vi "network2.vi"() -> ()   [LabVIEW 2009]
uses:
  <vilib>/vision/NI_Vision_Development_Module.lvlib
panel:
  out "Cluster":T1
  out "Filtered Image":T2(plugin-control)
  in  "res/2":i32
  in  "Sample Rate":i32=3
  out "Input Image":T2(plugin-control)
  in  "Input File Path":path
  in  "Stop Checking":bool
  out "Size of Inputs":i32
  in  "Num Iters":i32=2000
  out "Final Error":dbl(graph)
  in  "Stop Training":bool
  out "New Hidden Weights":dbl[][](array[numeric])
  out "Hidden Error":dbl[](array[numeric])
  out "New Output Weights":dbl[](array[numeric])
  in  "Training Constant":dbl=1.0
  out "Final Error for Back Prop":dbl
  out "Target":dbl
  out "Output":dbl
  in  "Num Not":i32=5
  in  "Num Line":i32=5
  out "Inputs":dbl[](array[numeric])
  in  "Num Hidden Layer":i32=128
  in  "Num Inputs":i32=64
  in  "Function Hidden Layer":u16(ring) items=["Siqmoid", "Linear", "Sign"]
  in  "Function Final Layer":u16(ring) items=["Siqmoid", "Linear", "Sign"]
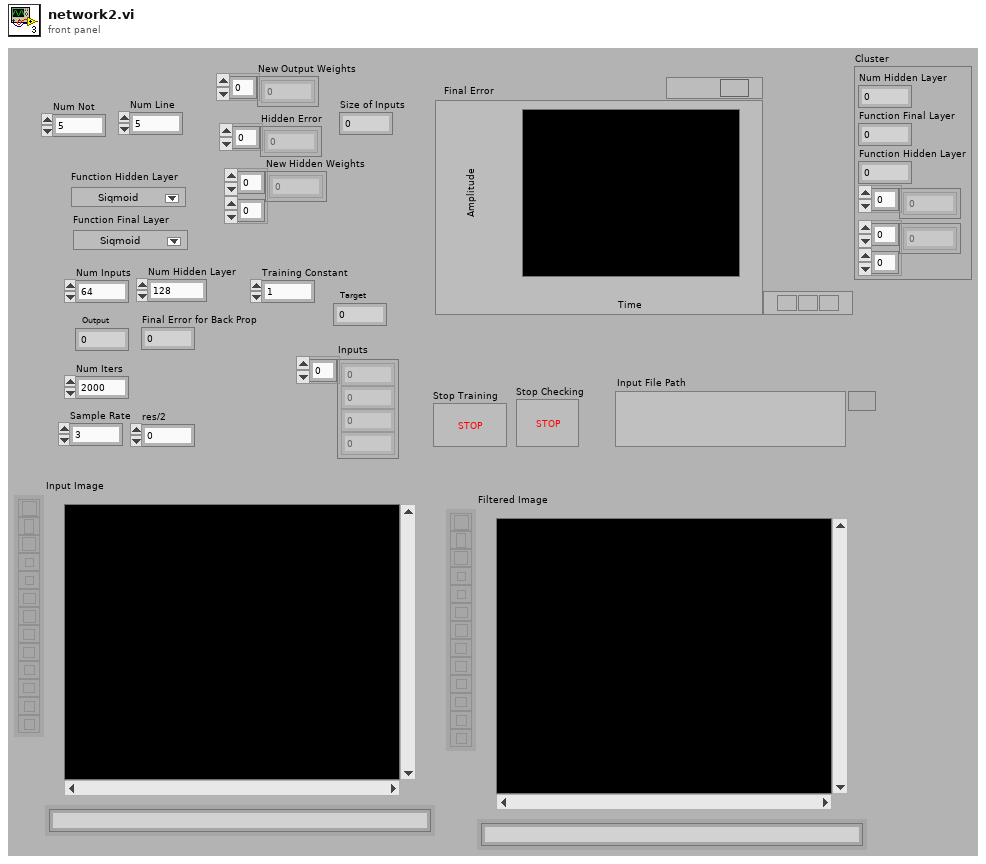
[diagram p1: front panel]
types:
  T1 = cluster{"Num Hidden Layer":i32, "Function Final Layer":u16, "Function Hidden Layer":u16, dbl[], dbl[][]}
  T2 = typedef "IMAQ Image.ctl" = refnum<image>
  T3 = typedef "Image Type" = u32
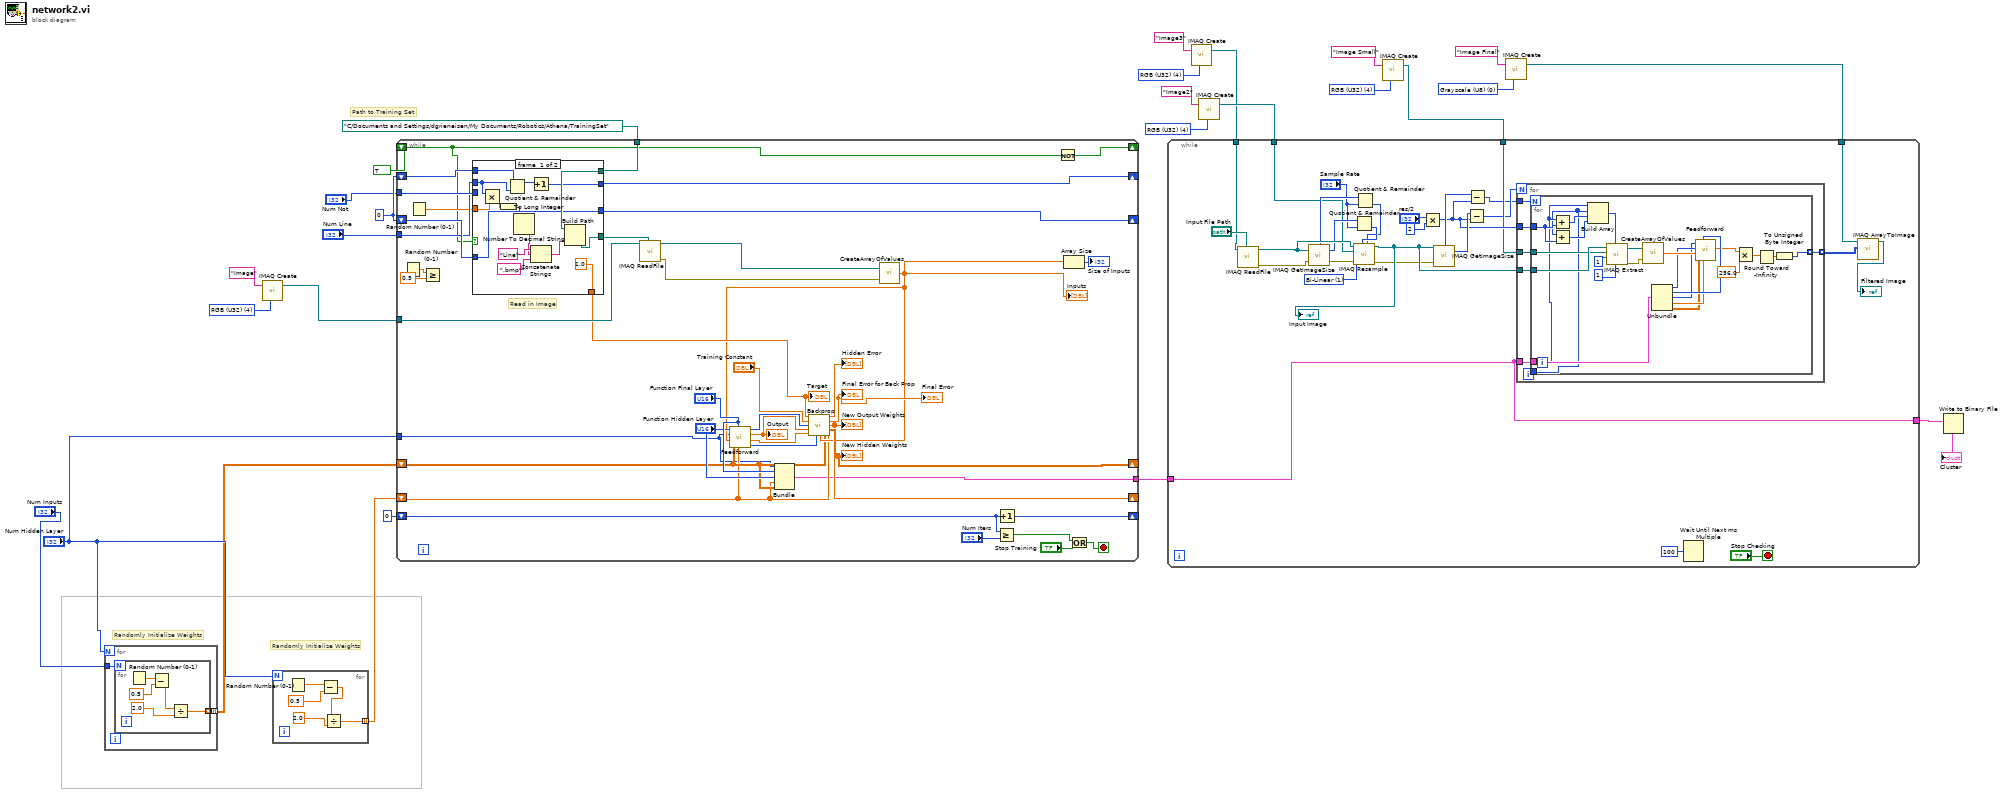
[diagram p0: block diagram]
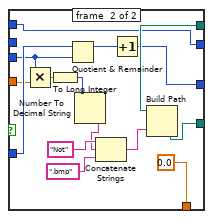
[diagram p2: hidden frame]
diagram:
  w4 = T3 4 items=["Grayscale (U8)", "Grayscale (I16)", "Grayscale (SGL)", "Complex (CSG)", "RGB (U32)", "HSL (U32)", "RGB (U64)", "Grayscale (U16)"] ("Image Type")
  w7 = T3 0 items=["Grayscale (U8)", "Grayscale (I16)", "Grayscale (SGL)", "Complex (CSG)", "RGB (U32)", "HSL (U32)", "RGB (U64)", "Grayscale (U16)"] ("Image Type")
  w11 = T3 4 items=["Grayscale (U8)", "Grayscale (I16)", "Grayscale (SGL)", "Complex (CSG)", "RGB (U32)", "HSL (U32)", "RGB (U64)", "Grayscale (U16)"] ("Image Type")
  w14 = T3 4 items=["Grayscale (U8)", "Grayscale (I16)", "Grayscale (SGL)", "Complex (CSG)", "RGB (U32)", "HSL (U32)", "RGB (U64)", "Grayscale (U16)"] ("Image Type")
  w21 = 0
  w25 = T3 4 items=["Grayscale (U8)", "Grayscale (I16)", "Grayscale (SGL)", "Complex (CSG)", "RGB (U32)", "HSL (U32)", "RGB (U64)", "Grayscale (U16)"] ("Image Type")
  # "Path to Training Set"
  # "Randomly Initialize Weights"
  # "Randomly Initialize Weights"
  n1 = for {
    N: "Num Hidden Layer" -> [_]
    tunnel: [w29] -> w22 mode=indexing
    tunnel: "Num Inputs" -> [w28]
    n2 = for {
      N: w28 -> [_]
      tunnel: [w30] -> w29 mode=indexing
      n3 = Random Number (0-1)() -> (number: 0 to 1=w31:dbl)
      n4 = Subtract(x=w31, y=0.5) -> (x-y=w33:dbl)
      n5 = Divide(x=w33, y=2.0) -> (x/y=w30:dbl)
    }
  }
  n6 = call "IMAQ Create"("Image Name"="Image", "Image Type"=w25) -> ("New Image"=w19:T2)  [unwired: 2 in, 2 out]
  n7 = for {
    N: "Num Hidden Layer" -> [_]
    tunnel: [w35] -> w23 mode=indexing
    n8 = Random Number (0-1)() -> (number: 0 to 1=w39:dbl)
    n9 = Subtract(x=w39, y=0.5) -> (x-y=w36:dbl)
    n10 = Divide(x=w36, y=2.0) -> (x/y=w35:dbl)
  }
  n11 = while {
    tunnel: "Num Hidden Layer" -> [w41]
    shift-right: [w73] -> _
    shift-left: w22 -> [w44]
    shift-right: [w72] -> _
    shift-left: w23 -> [w43]
    shift-right: [w52] -> _
    shift-left: w21 -> [w53]
    shift-right: [w55] -> _
    shift-left: w21 -> [w56]
    shift-right: [w71] -> _
    shift-left: TRUE -> [w40]
    tunnel: w19 -> [w70]
    tunnel: path "C:/Documents and Settings/dgrieneisen/My Documents/Robotics/Athena/TrainingSet" -> [w69]
    shift-right: [w60] -> _
    shift-left: 0 -> [w59]
    tunnel: "Num Not" -> [w57]
    tunnel: "Num Line" -> [w54]
    tunnel: [w42] -> w8
    stop <- w63 stop-if-true
    # "Read in Image"
    n12 = Random Number (0-1)() -> (number: 0 to 1=w50:dbl)
    n13 = Random Number (0-1)() -> (number: 0 to 1=w48:dbl)
    n14 = Greater Or Equal?(x=w50, y=0.5) -> ()  [unwired: 1 out]
    n15 = case shown="True" w40 {
      tunnel: w69 -> [w90 w105]
      tunnel: [w89 w104] -> w68
      tunnel: w53 -> [w85 w99]
      tunnel: w56 -> [w87 w101]
      tunnel: [1.0 0.0] -> w67
      tunnel: w57 -> [_ w95]
      tunnel: [w87 w102] -> w55
      tunnel: [w86 w99] -> w52
      tunnel: w54 -> [w80 _]
      tunnel: w48 -> [w81 w96]
      frame #0 {
        n16 = Multiply(x=w80, y=w81) -> (x*y=w83:dbl)
        n17 = To Long Integer(number=w83) -> (32bit integer=w82:i32)
        n18 = Quotient & Remainder(x=w85, y=w80) -> (x-y*floor(x/y)=w84:i32)  [unwired: 1 out]
        n19 = Number To Decimal String(number=w82) -> (decimal integer string=w92:string)  [unwired: 1 in]
        n20 = Increment(x=w84) -> (x+1=w86:i32)
        n21 = Concatenate Strings("Line", w92, ".bmp") -> (w94:string)
        n22 = Build Path(base path=w90, name or relative path=w94) -> (appended path=w89:path)
      }
      frame #1 {
        n23 = Multiply(x=w95, y=w96) -> (x*y=w98:dbl)
        n24 = To Long Integer(number=w98) -> (32bit integer=w97:i32)
        n25 = Quotient & Remainder(x=w101, y=w95) -> (x-y*floor(x/y)=w100:i32)  [unwired: 1 out]
        n26 = Number To Decimal String(number=w97) -> (decimal integer string=w107:string)  [unwired: 1 in]
        n27 = Concatenate Strings("Not", w107, ".bmp") -> (w109:string)
        n28 = Increment(x=w100) -> (x+1=w102:i32)
        n29 = Build Path(base path=w105, name or relative path=w109) -> (appended path=w104:path)
      }
    }
    "Target" <- w67
    n30 = call "IMAQ ReadFile"("File Path"=w68, "Image"=w70) -> ("error out"=w65:errorcluster, "Image Out"=w66:T2)  [unwired: 5 in, 3 out]
    n31 = Bundle("Num Hidden Layer"=w41, "Function Final Layer"="Function Final Layer", "Function Hidden Layer"="Function Hidden Layer", w43, w44) -> (w42:T1)  [unwired: 1 in]
    n32 = call "CreateArrayOfValues.vi"("error out"=w65, "Image Out"=w66) -> ("Array"=w45:dbl[])
    "Inputs" <- w45
    n33 = call "Feedforward.vi"("Final Weights"=w43, "Function Final Layer"="Function Final Layer", "Hidden Weights"=w44, "Inputs"=w45, "Num Hidden Layer"=w41, "Function Hidden Layer"="Function Hidden Layer") -> ("Function Hidden Layer 2"=w76:u16, "Hidden Outputs"=w77:dbl[], "Output"=w78:dbl, "Function Final Layer 2"=w79:u16)
    "Output" <- w78
    n34 = call "Backprop.vi"("Target"=w67, "Training Constant"="Training Constant", "Function Final Layer"=w79, "Output"=w78, "Hidden Outputs"=w77, "Function Hidden Layer"=w76, "Inputs"=w45, "Hidden Weights"=w44, "Final Weights"=w43) -> ("Hidden Error"=→"Hidden Error":dbl[], "Final Error for Back Prop"=→"Final Error for Back Prop" →"Final Error":dbl, "New Output Weights"=w72:dbl[], "New Hidden Weights"=w73:dbl[][])  [unwired: 3 in]
    "New Output Weights" <- w72
    "New Hidden Weights" <- w73
    n35 = Greater Or Equal?(x=w59, y="Num Iters") -> (x >= y?=w61:bool)
    n36 = Increment(x=w59) -> (x+1=w60:i32)
    n37 = Not(x=w40) -> (.not. x?=w71:bool)
    n38 = Array Size(array=w45) -> (size(s)=→"Size of Inputs":i32)
    n39 = Or(x=w61, y="Stop Training") -> (x .or. y?=w63:bool)
  }
  n40 = call "IMAQ Create"("Image Name"="Image3", "Image Type"=w11) -> ("New Image"=w9:T2)  [unwired: 2 in, 2 out]
  n41 = call "IMAQ Create"("Image Name"="Image2", "Image Type"=w14) -> ("New Image"=w12:T2)  [unwired: 2 in, 2 out]
  n42 = call "IMAQ Create"("Image Name"="Image Small", "Image Type"=w4) -> ("New Image"=w2:T2)  [unwired: 2 in, 2 out]
  n43 = call "IMAQ Create"("Image Name"="Image Final", "Image Type"=w7) -> ("New Image"=w5:T2)  [unwired: 2 in, 2 out]
  n44 = while {
    tunnel: w12 -> [w125]
    tunnel: w9 -> [w124]
    tunnel: w8 -> [w110]
    tunnel: w5 -> [w118]
    tunnel: w2 -> [w115]
    tunnel: [w110] -> w1
    stop <- "Stop Checking" stop-if-true
    w126 = u32 1 items=["Zero Order", "Bi-Linear", "Quadratic", "Cubic Spline"] ("Interpolation Type")
    n45 = call "IMAQ ReadFile"("File Path"="Input File Path", "Image"=w124) -> ("error out"=w134:errorcluster, "Image Out"=w133:T2)  [unwired: 5 in, 3 out]
    n46 = call "IMAQ GetImageSize"("Image"=w133, "error in (no error)"=w134) -> ("Y Resolution"=w130:i32, "X Resolution"=w131:i32, "error out"=w132:errorcluster)  [unwired: 2 in]
    n47 = Quotient & Remainder(x=w130, y="Sample Rate") -> (floor(x/y)=w129:i32)  [unwired: 1 out]
    n48 = Quotient & Remainder(x=w131, y="Sample Rate") -> (floor(x/y)=w128:i32)  [unwired: 1 out]
    n49 = call "IMAQ Resample"("X Resolution"=w128, "Y Resolution"=w129, "error in (no error)"=w132, "Interpolation Type"=w126, "Image Dst"=w125, "Image Src"=w133) -> ("error out"=w111:errorcluster, "Image Dst Out"=w116:T2)  [unwired: 4 in]
    "Input Image" <- w116
    n50 = Multiply(x="res/2", y=2) -> (x*y=w119:i32)
    n51 = call "IMAQ GetImageSize"("Image"=w116, "error in (no error)"=w111) -> ("Y Resolution"=w123:i32, "X Resolution"=w120:i32)  [unwired: 2 in, 1 out]
    n52 = Subtract(x=w123, y=w119) -> (x-y=w113:i32)
    n53 = Subtract(x=w120, y=w119) -> (x-y=w112:i32)
    n54 = for {
      N: w113 -> [_]
      tunnel: w119 -> [w144]
      tunnel: w116 -> [w143]
      tunnel: w110 -> [w142]
      tunnel: [w141] -> w114 mode=indexing
      tunnel: w115 -> [w140]
      tunnel: w112 -> [w139]
      i -> [w138]
      n55 = for {
        N: w139 -> [_]
        tunnel: w144 -> [w165]
        tunnel: w143 -> [w162]
        tunnel: w142 -> [w158]
        tunnel: [w148] -> w141 mode=indexing
        tunnel: w140 -> [w152]
        tunnel: w138 -> [w145]
        i -> [w146]
        n56 = Add(x=w146, y=w165) -> (x+y=w167:i32)
        n57 = Add(x=w145, y=w165) -> (x+y=w166:i32)
        n58 = Build Array(w146, w145, w167, w166) -> (w164:i32[])
        n59 = call "IMAQ Extract"("Y Step Size"=1, "Optional Rectangle"=w164, "X Step Size"=1, "Image Dst"=w152, "Image Src"=w162) -> ("error out"=w160:errorcluster, "Image Dst Out"=w161:T2)  [unwired: 1 in, 4 out]
        n60 = call "CreateArrayOfValues.vi"("error out"=w160, "Image Out"=w161) -> ("Array"=w159:dbl[])
        n61 = Unbundle(w158) -> ("Num Hidden Layer"=w157:i32, "Function Final Layer"=w156:u16, "Function Hidden Layer"=w155:u16, w154:dbl[], w153:dbl[][])
        n62 = call "Feedforward.vi"("Final Weights"=w154, "Function Final Layer"=w156, "Hidden Weights"=w153, "Inputs"=w159, "Num Hidden Layer"=w157, "Function Hidden Layer"=w155) -> ("Output"=w151:dbl)  [unwired: 3 out]
        n63 = Multiply(x=w151, y=256.0) -> (x*y=w149:dbl)
        n64 = Round Toward -Infinity(1:w149) -> (0:w147:dbl)
        n65 = To Unsigned Byte Integer(number=w147) -> (unsigned 8bit integer=w148:u8)
      }
    }
    n66 = Wait Until Next ms Multiple(millisecond multiple=u32 100) -> ()  [unwired: 1 out]
    n67 = call "IMAQ ArrayToImage"("Image Pixels (U8)"=w114, "Image"=w118) -> ("Image Out"=→"Filtered Image":T2)  [unwired: 8 in, 1 out]
  }
  "Cluster" <- w1
  n68 = Write to Binary File(data=w1) -> ()  [unwired: 5 in, 3 out]
